vi "GFM monitor.vi"() -> ()   [LabVIEW 2016, in "sub-VIs.lvlib"]
uses:
  sub-VIs/sub-VIs.lvlib
panel:
  in  "Reset data":bool
  in  "Acquisition Rate":enum32{"10 Hz", "1 Hz"}(radio)
  out "GFM field":dbl
  in  "stop":bool
  out "XY Graph":cluster{"X":dbl[], "Y":dbl[]}(graph)
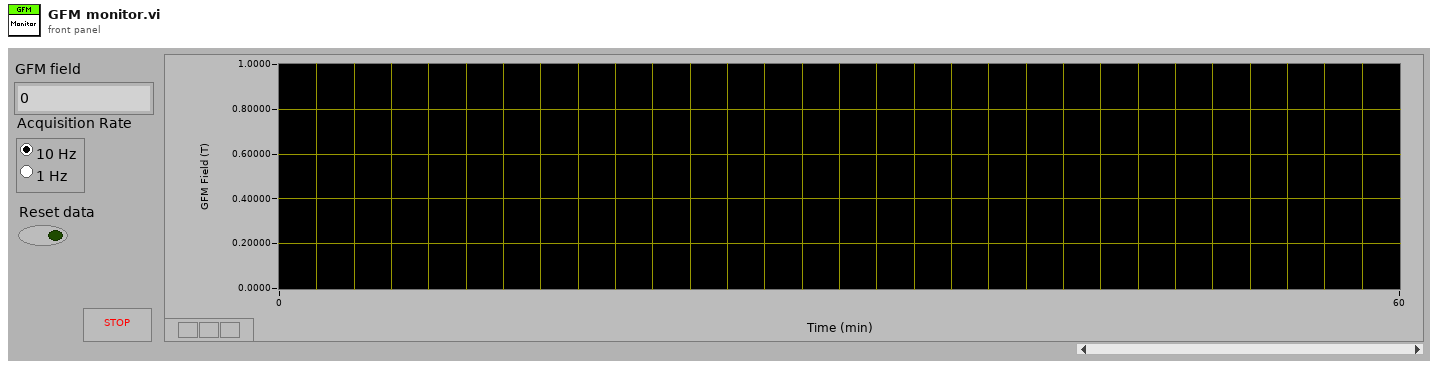
[diagram p1: front panel]
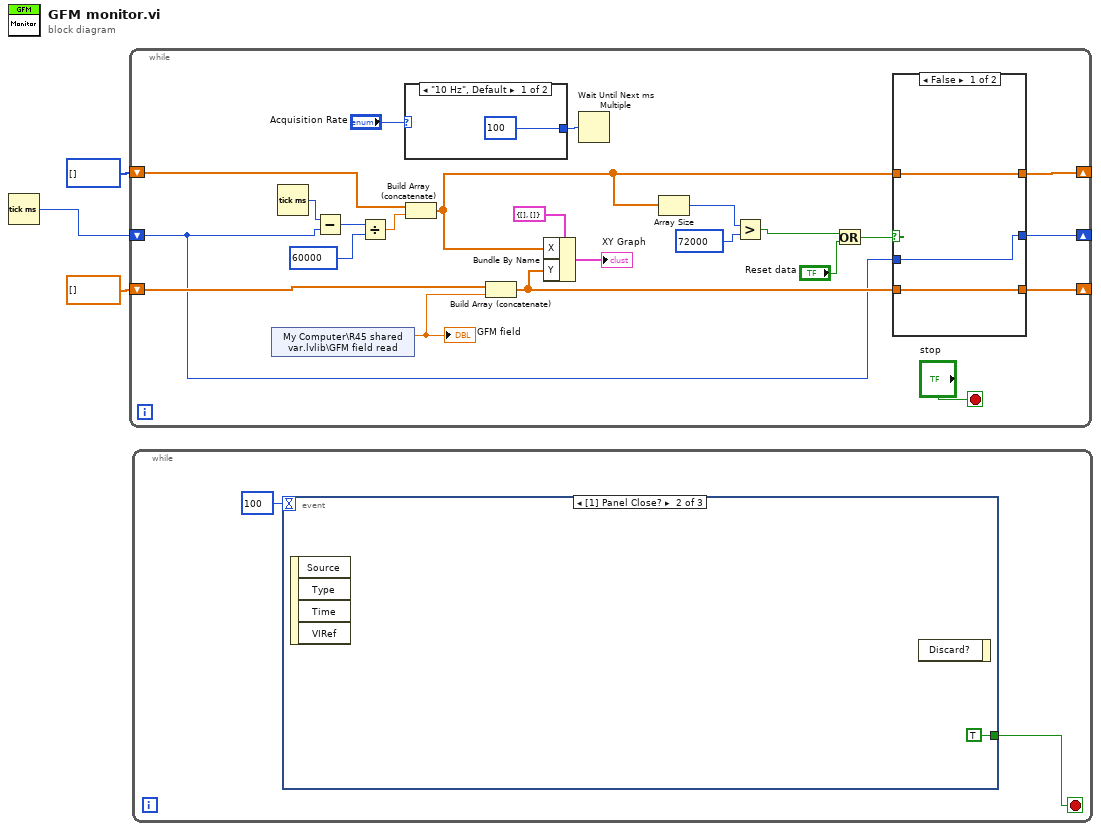
[diagram p0: block diagram]
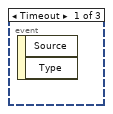
[diagram p2: hidden frame]
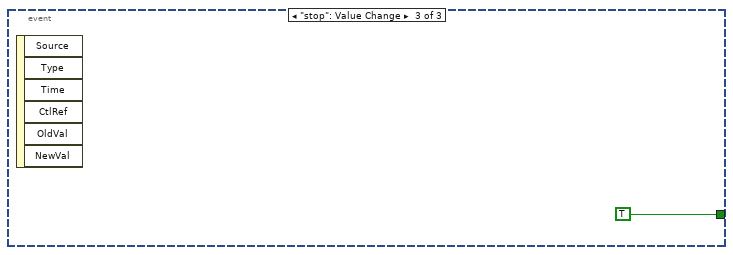
[diagram p3: hidden frame]
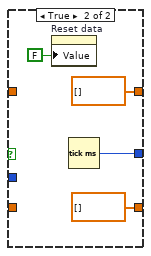
[diagram p4: hidden frame]
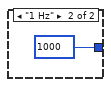
[diagram p5: hidden frame]
diagram:
  n1 = Tick Count (ms)() -> (millisecond timer value=w3:u32)
  n2 = while {
    shift-right: [w6] -> _
    shift-left: dbl[] [] -> [w24]
    shift-right: [w8] -> _
    shift-left: u32[] [] -> [w19]
    shift-right: [w5] -> _
    shift-left: w3 -> [w4]
    stop <- "stop" stop-if-true
    n3 = shared-variable "My Computer\\R45 shared var.lvlib\\GFM field read"() -> (w25:dbl)  [unwired: 1 in, 1 out]
    "GFM field" <- w25
    n4 = Tick Count (ms)() -> (millisecond timer value=w21:u32)
    n5 = Subtract(x=w21, y=w4) -> (x-y=w20:u32)
    n6 = Divide(x=w20, y=u32 60000) -> (x/y=w18:dbl)
    n7 = case shown="\"10 Hz\", Default" "Acquisition Rate" {
      tunnel: [100 1000] -> w15
      frame "10 Hz", Default {
      }
      frame "1 Hz" {
      }
    }
    n8 = Build Array (concatenate)(w19, w18) -> (w9:dbl[])
    n9 = Build Array (concatenate)(w24, w25) -> (w7:dbl[])
    n10 = Bundle By Name(cluster=cluster{"X":dbl[], "Y":dbl[]} {"X"=[], "Y"=[]} ("Cluster"), "X"=w9, "Y"=w7) -> (→"XY Graph":cluster{"X":dbl[], "Y":dbl[]})
    n11 = Wait Until Next ms Multiple(millisecond multiple=w15) -> ()  [unwired: 1 out]
    n12 = Array Size(array=w9) -> (size(s)=w14:i32)
    n13 = Greater?(x=w14, y=72000) -> (0:w12:bool)
    n14 = Or(x=w12, y="Reset data") -> (x .or. y?=w10:bool)
    n15 = case shown="False" w10 {
      tunnel: w9 -> [w29 _]
      tunnel: [w29 dbl[] []] -> w8
      tunnel: w7 -> [w28 _]
      tunnel: [w28 dbl[] []] -> w6
      tunnel: [w27 w30] -> w5
      tunnel: w4 -> [w27 _]
      frame False {
      }
      frame True {
        n16 = property on="Reset data" class="Bool (strict)"("Value"=FALSE ("Reset data")) -> ()  [unwired: 2 in, 2 out]
        n17 = Tick Count (ms)() -> (millisecond timer value=w30:u32)
      }
    }
  }
  n18 = while {
    stop <- w37 stop-if-true
    n19 = event shown="[1] Panel Close?" {
      selector: _ -> [_ _ _]
      dyn-events: _ -> [_ _ _]
      timeout: 100 -> [_ _ _]
      tunnel: [_ TRUE TRUE] -> w37
      event Timeout {
        n20 = event-data() -> ()  [unwired: 1 in, 2 out]
      }
      event Panel Close? {
        n21 = event-data() -> ()  [unwired: 1 in, 4 out]
        n22 = event-data() -> ()  [unwired: 2 in, 1 out]
      }
      event "stop": Value Change {
        n23 = event-data() -> ()  [unwired: 1 in, 6 out]
      }
    }
  }
